vi "setAmount.vi"(8 "error in (no error)":errorcluster, 10 "Amount":dbl, 11 "Goal in":refnum<class "Goal.lvclass">) -> (0 "error out":errorcluster, 3 "Goal out":refnum<class "Goal.lvclass">)   [LabVIEW 2018, in "Goal.lvclass"]
uses:
  Goal.lvclass
  Goal.lvclass/Goal.ctl
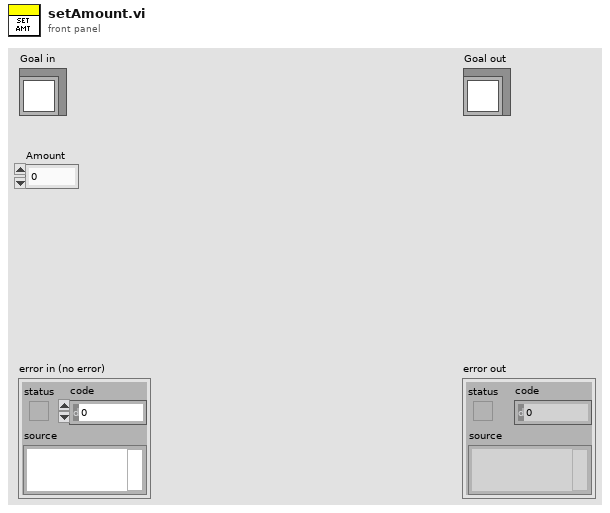
[diagram p1: front panel]
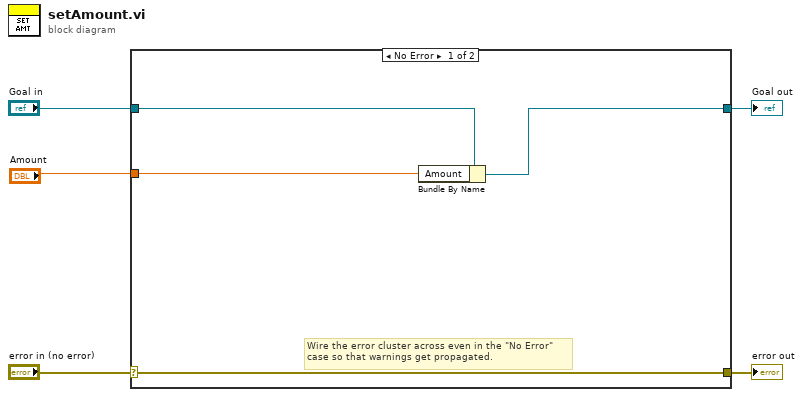
[diagram p0: block diagram]
diagram:
  n1 = case shown="No Error" "error in (no error)" {
    selector: "error in (no error)" -> [w9 w11]
    tunnel: [w9 w11] -> w4
    tunnel: [w7 w10] -> w2
    tunnel: "Goal in" -> [w8 w10]
    tunnel: "Amount" -> [w6 _]
    frame No Error {
      # "Wire the error cluster across even in the \"No Error\"\ncase so that warnings get propagated."
      n2 = Bundle By Name(cluster=w8, "Amount"=w6) -> (w7:refnum<class "Goal.lvclass">)
    }
    frame Error {
    }
  }
  "error out" <- w4
  "Goal out" <- w2
